vi "Main_04A.vi"() -> ()   [LabVIEW 2024]
uses:
  TypeDefs/Cluster Row-Column.ctl
panel:
  out "Answer 2569":u32
  in  "Puzzle":string="XXASMSMSXMXSMMXMAXMMMAMSAMASMSAMXMAXSXMASMAMMXXMASASXAMAMXSXMMSXSAMXSSXXMXAAXMAXMXXSXMXMMAAMMMMMMMMMMXXMSMSSSMXAAMAMMMSAMXXXXSMSAXMMXXMASMSS\nASMMAAAMAMASAXSSMMSASAMXAAAAXXXMAXXAMSASXMASMSSMSAMSAMMSXMAXSMAAMMSAMAAMSMSMSSSSXSXSMSAAXMXMAAAAMMSAMXSXMAAAAAXMAMAMAMAMMXMSASAXMXSAMXSAMXAS\nXSAMSMMSAMASXMXAAXSASXXSSMXXXMMSMSMSMAMMASASXAAXXAMXAXAMAXMASMMSMAMMSMSMAAAAAAAAASASASXSMSASXSSXSAXAMAMAMMMSMMMMAXASMSMXSAAMAMXMMAMAXXAMXMMS\nAMAMXAASMMXSAMSMMMMMMMMMAMMSMMAAAAAAXAXSAMASMSSMSAMSAMMSMMMXXAAAMXMAAAAMXMMMMSMMMMAMAMAMAMMSXMAXMASXMSSMSAMXAAASMSMXAAXAMMSMAAMAMXSMMSASXSXM\nXSAMMMMXAXSMXXAMAAXSAAXSAMASAAMMSMSM..."
  in  "Example":string="MMMSXXMASM\nMSAMXMSMSA\nAMXSXMAAMM\nMSAMASMSMX\nXMASAMXAMM\nXXAMMXXAMA\nSMSMSASXSS\nSAXAMASAAA\nMAMMMXMMMM\nMXMXAXMASX"
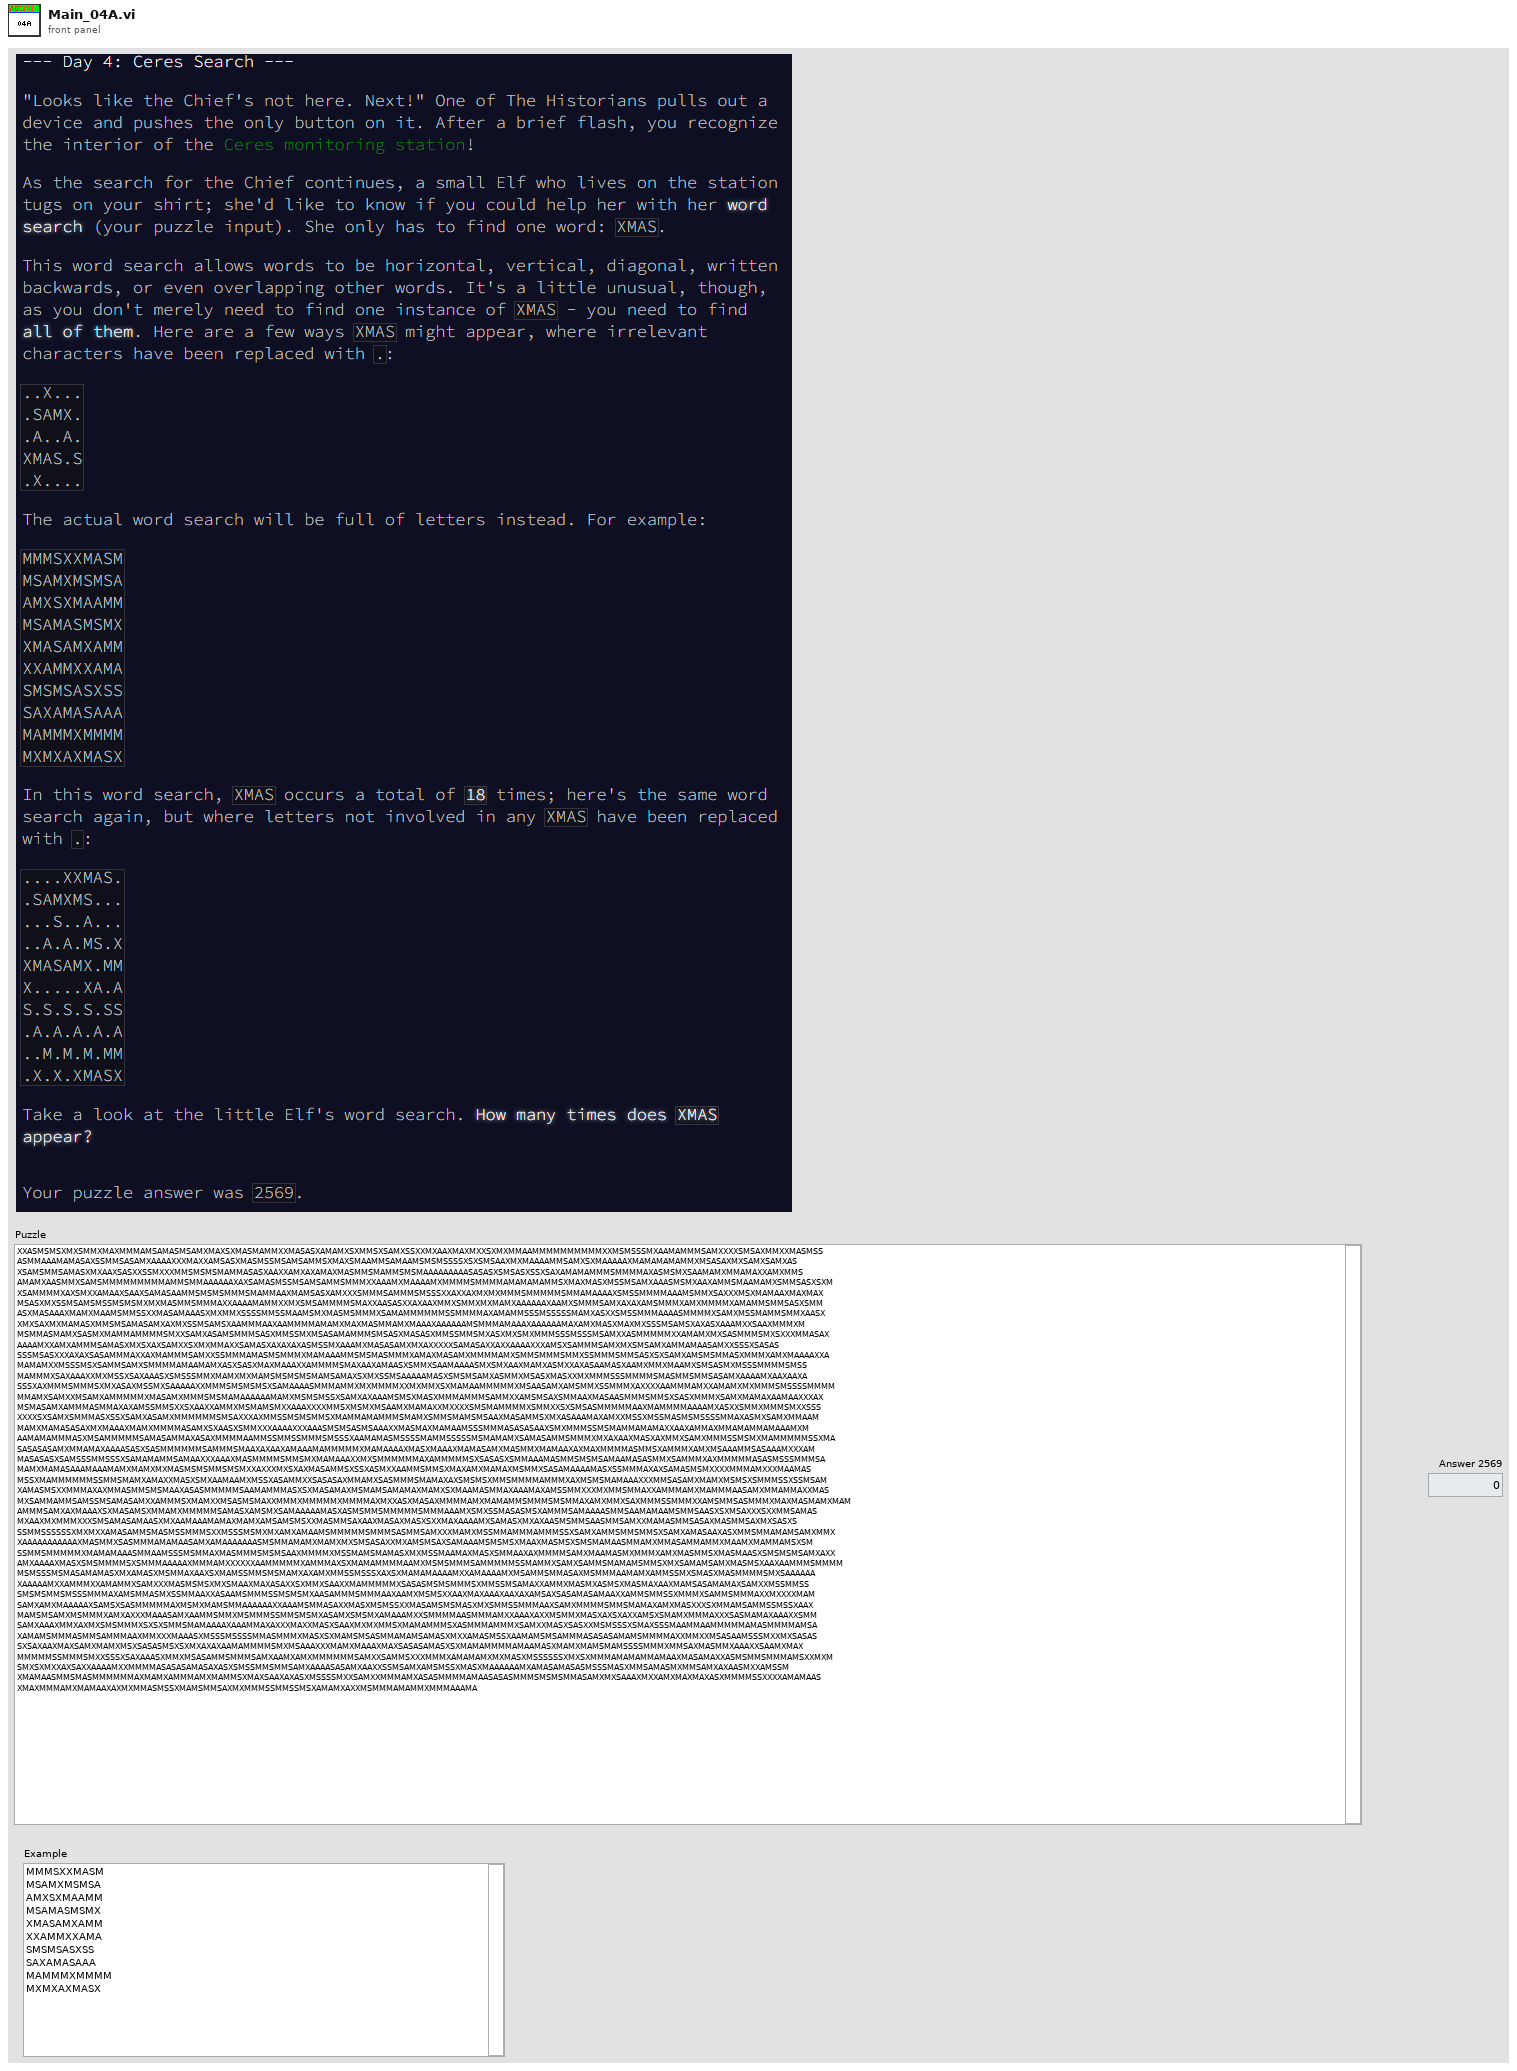
[diagram p1: front panel]
types:
  T1 = typedef "Cluster Row-Column.ctl" = cluster{"R":i32, "C":i32}
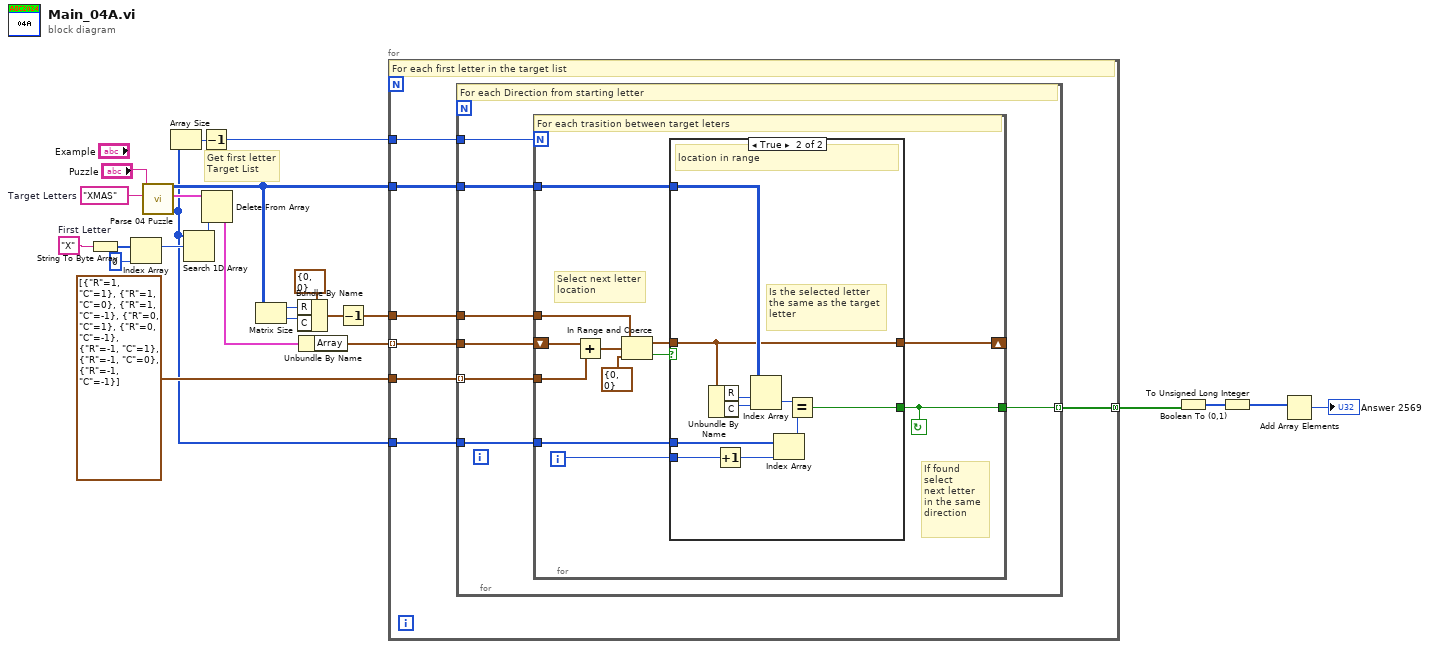
[diagram p0: block diagram]
diagram:
  w8 = "X"  # First Letter
  w24 = "XMAS"  # Target Letters
  # "Get first letter\nTarget List"
  n1 = String To Byte Array(string=w8) -> (unsigned byte array=w7:u8[])
  n2 = Index Array(array=w7, index=0) -> (element=w5:u8)
  n3 = call "Parse 04 Puzzle.vi"("Target Letters"=w24, "Puzzle"="Puzzle") -> ("Axcii Target Letters Out"=w3:u8[], "Letter Location Array Out"=w23:cluster{"Array":T1[]}[], "Ascii Byte Array Out"=w20:u8[][])  [unwired: 7 in]
  n4 = Array Size(array=w3) -> (size(s)=w2:i32)
  n5 = Search 1D Array(1D array=w3, element=w5) -> (index of element=w4:i32)  [unwired: 1 in]
  n6 = Decrement(x=w2) -> (x-1=w1:i32)
  n7 = Delete From Array(array=w23, index=w4) -> (deleted portion=w22:cluster{"Array":T1[]})  [unwired: 1 in, 1 out]
  n8 = Matrix Size(0:w20) -> (1:w17:i32, 2:w16:i32)
  n9 = Bundle By Name(cluster=T1 {"R"=0, "C"=0}, "R"=w17, "C"=w16) -> (w15:T1)
  n10 = Unbundle By Name(w22) -> ("Array"=w21:T1[])
  n11 = Decrement(x=w15) -> (x-1=w14:T1)
  n12 = for {
    tunnel: w21 -> [w27] mode=indexing
    tunnel: w20 -> [w31]
    tunnel: T1[] [{"R"=1, "C"=1}, {"R"=1, "C"=0}, {"R"=1, "C"=-1}, {"R"=0, "C"=1}, {"R"=0, "C"=-1}, {"R"=-1, "C"=1}, {"R"=-1, "C"=0}, {"R"=-1, "C"=-1}] -> [w29]
    tunnel: w14 -> [w28]
    tunnel: w3 -> [w30]
    tunnel: [w26] -> w12 mode=concatenating
    tunnel: w1 -> [w25]
    # "For each first letter in the target list"
    n13 = for {
      tunnel: w31 -> [w38]
      tunnel: w28 -> [w34]
      tunnel: w30 -> [w37]
      tunnel: w29 -> [w35] mode=indexing
      tunnel: [w33] -> w26 mode=indexing
      tunnel: w27 -> [w36]
      tunnel: w25 -> [w32]
      # "For each Direction from starting letter"
      n14 = for {
        N: w32 -> [_]
        tunnel: w38 -> [w50]
        tunnel: w37 -> [w49]
        tunnel: w35 -> [w46]
        tunnel: w34 -> [w43]
        tunnel: [w39] -> w33
        shift-right: [w41] -> _
        shift-left: w36 -> [w47]
        i -> [w40]
        stop <- w39 continue-if-true
        # "If found\nselect\nnext letter\nin the same \ndirection"
        # "Select next letter\nlocation"
        # "For each trasition between target leters"
        n15 = Add(x=w47, y=w46) -> (x+y=w48:T1)
        n16 = In Range and Coerce(upper limit=w43, x=w48, lower limit=T1 {"R"=0, "C"=0}) -> (coerced(x)=w44:T1, In Range?=w42:bool)
        n17 = case shown="True" w42 {
          selector: w42 -> [w52 _]
          tunnel: w50 -> [_ w62]
          tunnel: w49 -> [_ w61]
          tunnel: w44 -> [w51 w53]
          tunnel: w40 -> [_ w55]
          tunnel: [w52 w54] -> w39
          tunnel: [w51 w53] -> w41
          frame False {
            # "location NOT in range"
          }
          frame True {
            # "Is the selected letter\nthe same as the target\nletter"
            # "location in range"
            n18 = Unbundle By Name(w53) -> ("R"=w60:i32, "C"=w59:i32)
            n19 = Increment(x=w55) -> (x+1=w57:i32)
            n20 = Index Array(array=w62, index (row)=w60, index (col)=w59) -> (element=w58:u8)
            n21 = Index Array(array=w61, index=w57) -> (element=w56:u8)
            n22 = Equal?(x=w58, y=w56) -> (x = y?=w54:bool)
          }
        }
      }
    }
  }
  n23 = Boolean To (0,1)(Boolean=w12) -> (0, 1=w11:i16[])
  n24 = To Unsigned Long Integer(number=w11) -> (unsigned 32bit integer=w10:u32[])
  n25 = Add Array Elements(numeric array=w10) -> (sum=→"Answer 2569":u32)
